vi "OutputDialog.vi"() -> (3 "Cancelled?":bool)   [LabVIEW 2020]
doc: "Use this template to create a dialog box with event handling."
uses:
  global/SettingVariable.vi
  <vilib>/Utility/config.llb/Write Key (Boolean).vi
  <vilib>/Utility/config.llb/Write Key (U32).vi
  <vilib>/Utility/config.llb/Write Key (I32).vi
  <vilib>/Utility/config.llb/Write Key (Double).vi
  <vilib>/Utility/config.llb/NI_LVConfig.lvlib
panel:
  in  "输出电压控件组":T1(array[cluster])=[{"开关"=FALSE, "输出选择"=0, "电压范围"={"Numeric"=5, "Numeric"=1}, "线性/对数"=FALSE, "物理量上限"=100.0, "物理量下限"=-100.0}, {"开关"=FALSE, "输出选择"=0, "电压范围"={"Numeric"=5, "Numeric"=1}, "线性/对数"=FALSE, "物理量上限"=100.0, "物理量下限"=-100.0}, {"开关"=FALSE, "输出选择"=0, "电压范围"={"Numeric"=5, "Numeric"=1}, "线性/对数"=FALSE, "物理量上限"=100.0, "物理量下限"=-100.0}, {"开关"=FALSE, "输出选择"=0, "电压范围"={"Numeric"=5, "Numeric"=1}, "线性/对数"=FALSE, "物理量上限"=100.0, "物理量下限"=-100.0}] {"电压范围" scale=-10.0..10.0; "输出选择" items=["电流1", "电流1反应性", "电流2", "电流2反应性"]}
  out "电流输入指示":bool[](array[boolean])
  out "电压标尺指示":u16[](array[ring]) items=["计数通量", "电压通量", "电流通量", "棒位", "温度", "P2参数", "硼浓度"]
  out "电压输入指示":bool[](array[boolean])
  in  "Cancel":bool
  in  "OK":bool
  # "输入状态"
  # "输出电压设置"
  # "输出电压1："
  # "输出电压2："
  # "输出电压3："
  # "输出电压4："
  # "电流1"
  # "电流2"
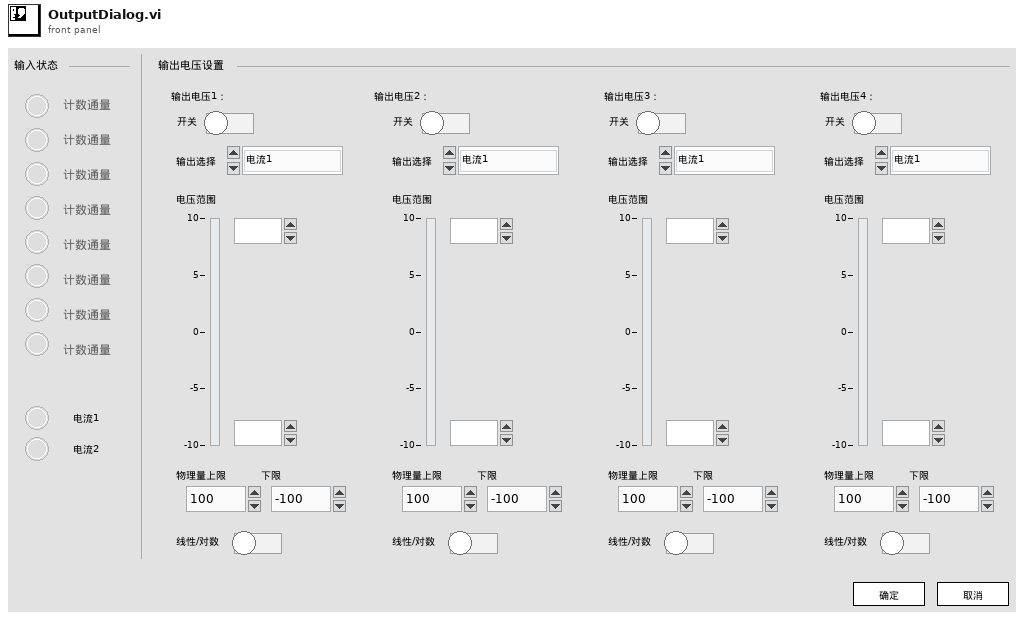
[diagram p1: front panel]
types:
  T1 = cluster{"开关":bool, "输出选择":u16, "电压范围":cluster{"Numeric":i32, "Numeric":i32}, "线性/对数":bool, "物理量上限":dbl, "物理量下限":dbl}[]
  T2 = cluster{"switch":bool, "voltage upper":i32, "voltage lower":i32, "physics upper":dbl, "physics lower":dbl, "input":u16, "log":bool}[]
  T3 = cluster{"switch":bool, "name":string, "voltage upper":i32, "voltage lower":i32, "physics upper":dbl, "physics lower":dbl, "scale":u16}[]
  T4 = cluster{"开关":bool, "输出选择":u16, "电压范围":cluster{"Numeric":i32, "Numeric":i32}, "线性/对数":bool, "物理量上限":dbl, "物理量下限":dbl}
  T5 = enum16{"fractional", "engineering", "exponential"}
  T6 = typedef "NI_LVConfig.lvlib/Config Data RefNum.ctl" = refnum<k1>
  T7 = cluster{"switch":bool, "voltage upper":i32, "voltage lower":i32, "physics upper":dbl, "physics lower":dbl, "input":u16, "log":bool}
  T8 = cluster{"开关":bool, "输出选择":bool, "电压范围":cluster{"Numeric":bool, "Numeric":bool}, "线性/对数":bool, "物理量上限":bool, "物理量下限":bool}[]
  T9 = enum32{"Bad", "Idle", "Run top level", "Running"}
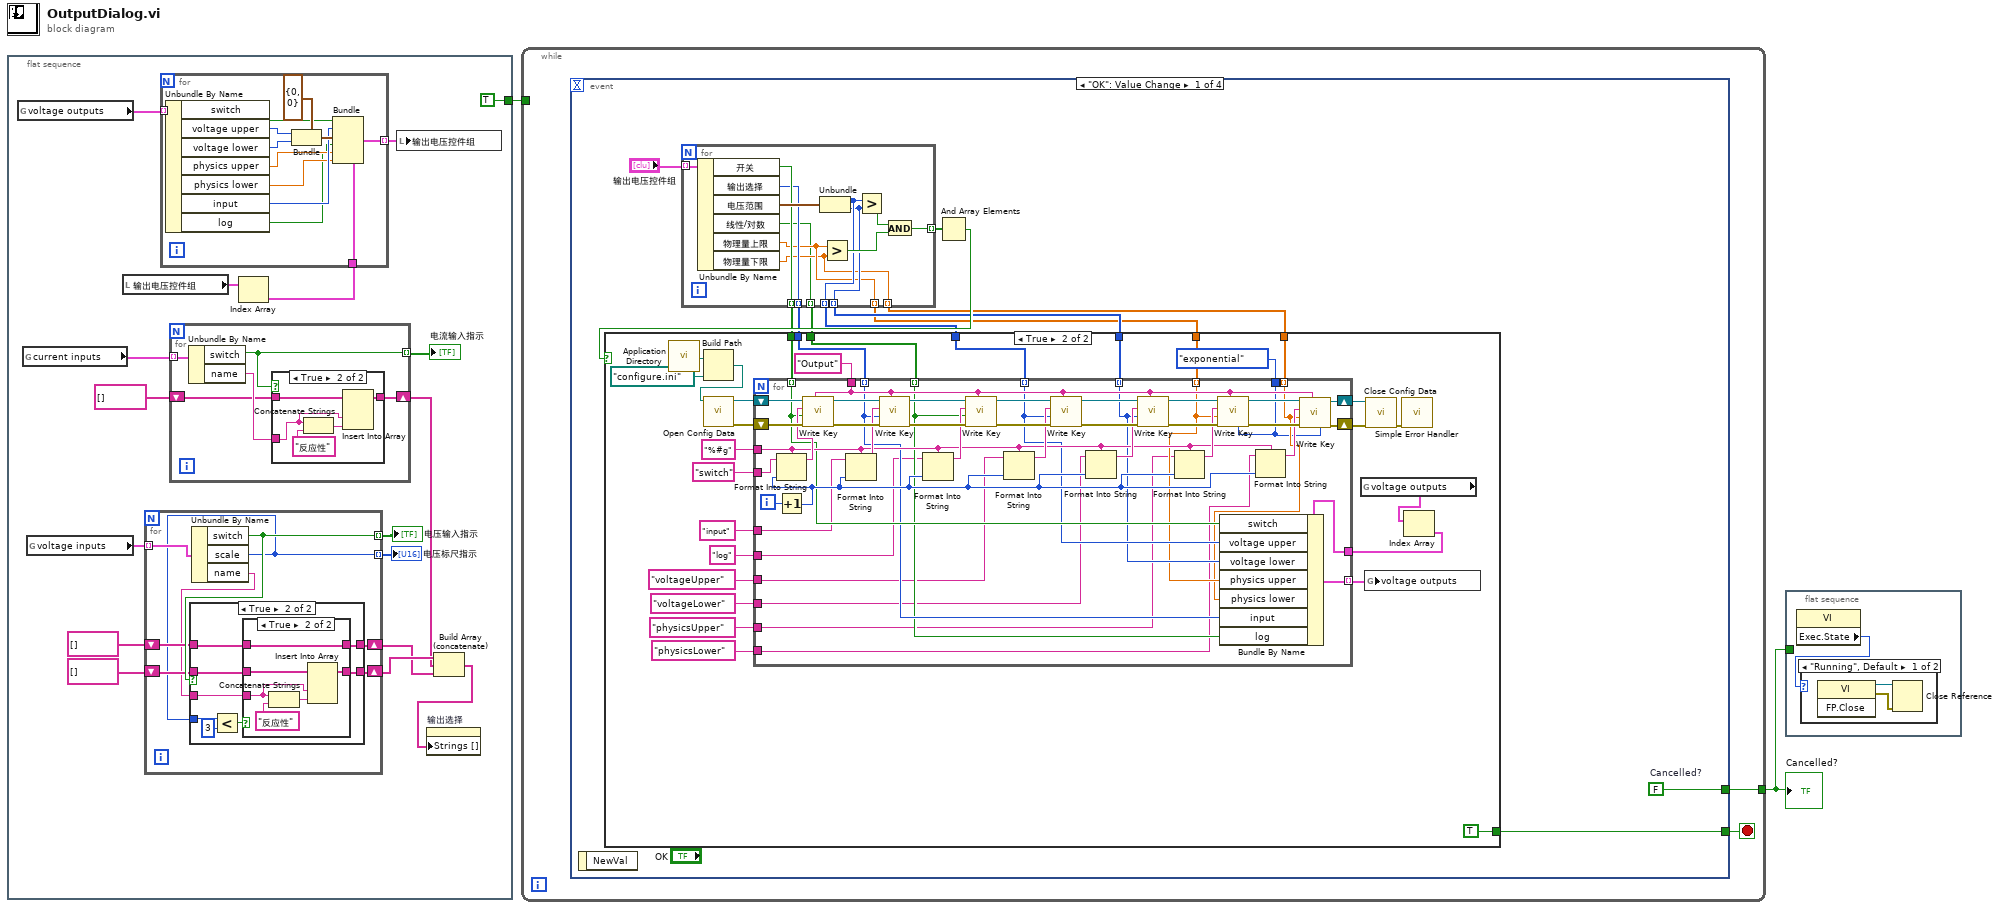
[diagram p0: block diagram]
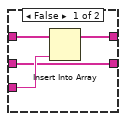
[diagram p4: hidden frame]
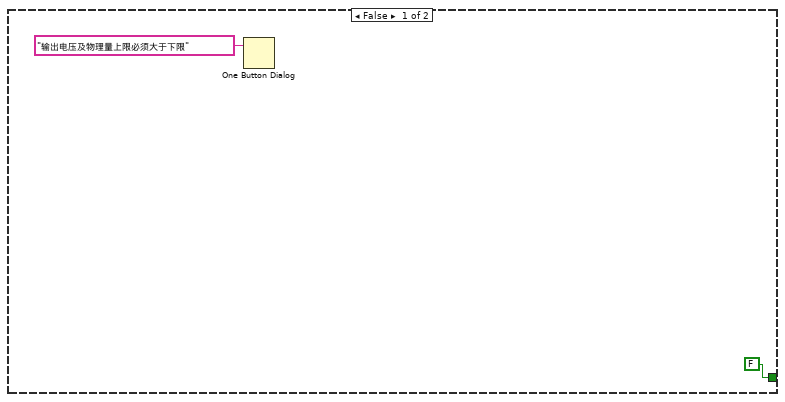
[diagram p6: hidden frame]
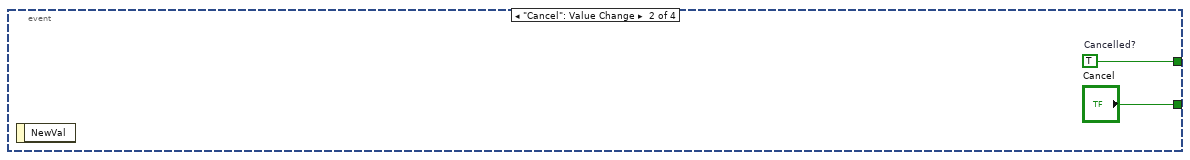
[diagram p7: hidden frame]
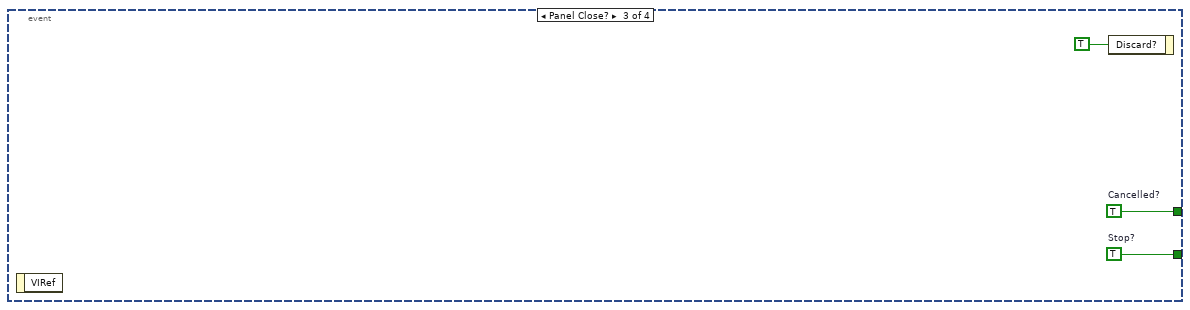
[diagram p8: hidden frame]
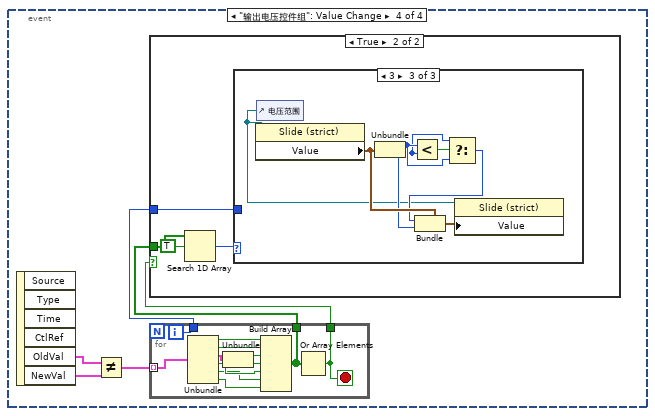
[diagram p9: hidden frame]
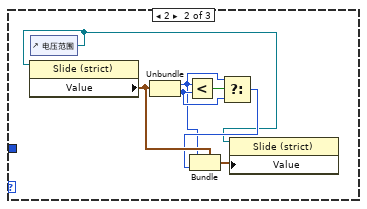
[diagram p12: hidden frame]
diagram:
  n1 = flat-sequence {
    tunnel: [TRUE] -> w2
    frame #0 {
      n2 = global read "SettingVariable.vi" "voltage outputs"() -> (w14:T2)
      n3 = global read "SettingVariable.vi" "current inputs"() -> (w19:cluster{"name":string, "switch":bool}[])
      n4 = global read "SettingVariable.vi" "voltage inputs"() -> (w17:T3)
      n5 = local read "输出电压控件组"() -> (w13:T1)
      n6 = for {
        tunnel: w17 -> [w39] mode=indexing
        tunnel: [w38] -> w16 mode=indexing
        tunnel: [w32] -> w15 mode=indexing
        shift-right: [w36] -> w6
        shift-left: string[] [] ("子数组") -> [w37]
        shift-right: [w34] -> w4
        shift-left: string[] [] ("子数组") -> [w35]
        n7 = Unbundle By Name(w39) -> ("switch"=w38:bool, "scale"=w32:u16, "name"=w33:string)
        n8 = case shown="True" w38 {
          tunnel: w37 -> [w41 w46]
          tunnel: w32 -> [_ w49]
          tunnel: [w41 w45] -> w36
          tunnel: w33 -> [_ w44]
          tunnel: w35 -> [w40 w42]
          tunnel: [w40 w43] -> w34
          frame False {
          }
          frame True {
            n9 = Less?(x=w49, y=u16 3) -> (x < y?=w47:bool)
            n10 = case shown="True" w47 {
              tunnel: w46 -> [w50 w57]
              tunnel: [w50 w56] -> w45
              tunnel: w44 -> [w53 w55]
              tunnel: [w51 w54] -> w43
              tunnel: w42 -> [w52 w54]
              frame False {
                n11 = Insert Into Array(array=w52, new element=w53) -> (w51:string[])  [unwired: 1 in]
              }
              frame True {
                n12 = Concatenate Strings(w55, "反应性" ("字符串")) -> (w58:string)
                n13 = Insert Into Array(array=w57, new element #1=w55, new element #2=w58) -> (w56:string[])  [unwired: 1 in]
              }
            }
          }
        }
      }
      "电压输入指示" <- w16
      "电压标尺指示" <- w15
      n14 = for {
        tunnel: w19 -> [w64] mode=indexing
        tunnel: [w63] -> w18 mode=indexing
        shift-right: [w61] -> w5
        shift-left: string[] [] -> [w60]
        n15 = Unbundle By Name(w64) -> ("switch"=w63:bool, "name"=w62:string)
        n16 = case shown="True" w63 {
          tunnel: w60 -> [w65 w70]
          tunnel: [w65 w69] -> w61
          tunnel: w62 -> [_ w66]
          frame False {
          }
          frame True {
            n17 = Concatenate Strings(w66, "反应性" ("字符串")) -> (w67:string)
            n18 = Insert Into Array(array=w70, new element #1=w66, new element #2=w67) -> (w69:string[])  [unwired: 1 in]
          }
        }
      }
      "电流输入指示" <- w18
      n19 = Index Array(array=w13) -> (element=w12:T4)  [unwired: 1 in]
      n20 = for {
        tunnel: w14 -> [w31] mode=indexing
        tunnel: w12 -> [w27]
        tunnel: [w20] -> w11 mode=indexing
        n21 = Unbundle By Name(w31) -> ("switch"=w24:bool, "voltage upper"=w29:i32, "voltage lower"=w28:i32, "physics upper"=w23:dbl, "physics lower"=w22:dbl, "input"=w25:u16, "log"=w21:bool)
        n22 = Bundle(cluster=cluster{i32, i32} {0, 0}, w29, w28) -> (w26:cluster{i32, i32})
        n23 = Bundle(cluster=w27, "开关"=w24, "输出选择"=w25, "电压范围"=w26, "线性/对数"=w21, "物理量上限"=w23, "物理量下限"=w22) -> (w20:T4)
      }
      n24 = local write "输出电压控件组"(w11) -> ()
      n25 = Build Array (concatenate)(w6, w5, w4) -> (w3:string[])
      n26 = property on="输出选择" class="Ring (strict)"("Strings []"=w3) -> ()  [unwired: 2 in, 2 out]
    }
  }
  n27 = while {
    tunnel: [w71] -> w1
    tunnel: w2 -> [_]
    stop <- w72 stop-if-true
    n28 = event shown="[0] \"OK\": Value Change" {
      selector: _ -> [_ _ _ _]
      dyn-events: _ -> [_ _ _ _]
      timeout: _ -> [_ _ _ _]
      tunnel: [w73 "Cancel" w175 _] -> w72
      tunnel: [w84 w173 w174 _] -> w71
      event "OK": Value Change {
        w84 = FALSE  # Cancelled?
        n29 = event-data() -> ()  [unwired: 1 in, 1 out]
        n30 = for {
          tunnel: "输出电压控件组" -> [w171] mode=indexing
          tunnel: [w167] -> w82 mode=indexing
          tunnel: [w166] -> w80 mode=indexing
          tunnel: [w165] -> w79 mode=indexing
          tunnel: [w164] -> w77 mode=indexing
          tunnel: [w163] -> w76 mode=indexing
          tunnel: [w162] -> w75 mode=indexing
          tunnel: [w161] -> w74 mode=indexing
          tunnel: [w160] -> w78 mode=indexing
          n31 = Unbundle By Name(w171) -> ("开关"=w166:bool, "输出选择"=w165:u16, "电压范围"=w170:cluster{"Numeric":i32, "Numeric":i32}, "线性/对数"=w160:bool, "物理量上限"=w162:dbl, "物理量下限"=w161:dbl)
          n32 = Unbundle(w170) -> ("Numeric"=w164:i32, "Numeric"=w163:i32)
          n33 = Greater?(x=w162, y=w161) -> (0:w168:bool)
          n34 = Greater?(x=w164, y=w163) -> (0:w169:bool)
          n35 = And(x=w169, y=w168) -> (x .and. y?=w167:bool)
        }
        n36 = And Array Elements(Boolean array=w82) -> (logical AND=w81:bool)
        n37 = case shown="True" w81 {
          tunnel: w80 -> [_ w115]
          tunnel: w79 -> [_ w103]
          tunnel: w78 -> [_ w102]
          tunnel: w77 -> [_ w101]
          tunnel: w76 -> [_ w100]
          tunnel: w75 -> [_ w99]
          tunnel: w74 -> [_ w98]
          tunnel: [FALSE ("Stop?") TRUE ("Stop?")] -> w73
          frame False {
            n38 = One Button Dialog(message="输出电压及物理量上限必须大于下限") -> ()  [unwired: 1 in, 1 out]
          }
          frame True {
            n39 = call <vilib>:"Application Directory.vi"() -> ("Application Directory"=w114:path)
            n40 = Build Path(base path=w114, name or relative path=path "configure.ini") -> (appended path=w112:path)
            n41 = call <vilib>:"Open Config Data.vi"("configuration file path"=w112) -> ("error out"=w110:errorcluster, "refnum"=w111:T6)  [unwired: 2 in, 7 out]
            n42 = global read "SettingVariable.vi" "voltage outputs"() -> (w96:T2)
            n43 = Index Array(array=w96) -> (element=w95:T7)  [unwired: 1 in]
            n44 = for {
              tunnel: w115 -> [w129] mode=indexing
              tunnel: "Output" ("section") -> [w137]
              tunnel: "%#g" ("section") -> [w132]
              tunnel: "switch" ("initial string") -> [w156]
              shift-right: [w142] -> w104
              shift-left: w110 -> [w158]
              shift-right: [w143] -> w105
              shift-left: w111 -> [w159]
              tunnel: w103 -> [w128] mode=indexing
              tunnel: w102 -> [w127] mode=indexing
              tunnel: w101 -> [w126] mode=indexing
              tunnel: w100 -> [w125] mode=indexing
              tunnel: w99 -> [w124] mode=indexing
              tunnel: w98 -> [w123] mode=indexing
              tunnel: [w131] -> w97 mode=indexing
              tunnel: w95 -> [w130]
              tunnel: "input" ("initial string") -> [w122]
              tunnel: "log" ("initial string") -> [w121]
              tunnel: "voltageUpper" ("initial string") -> [w120]
              tunnel: "voltageLower" ("initial string") -> [w119]
              tunnel: "physicsUpper" ("initial string") -> [w118]
              tunnel: "physicsLower" ("initial string") -> [w117]
              tunnel: T5."exponential" ("format (fractional)") -> [w116]
              i -> [w157]
              n45 = Increment(x=w157) -> (x+1=w133:i32)
              n46 = Format Into String(format string=w132, initial string=w156, w133) -> (resulting string=w155:string)  [unwired: 1 in, 1 out]
              n47 = call-poly <vilib>:"Write Key.vi"("section"=w137, "error in (no error)"=w158, "value"=w129, "key"=w155, "refnum"=w159) -> ("error out"=w154:errorcluster, "refnum out"=w153:T6)  [unwired: 4 in, 1 out]
              n48 = Format Into String(format string=w132, initial string=w122, w133) -> (resulting string=w148:string)  [unwired: 1 in, 1 out]
              n49 = call-poly <vilib>:"Write Key.vi"("section"=w137, "error in (no error)"=w154, "value"=w128, "key"=w148, "refnum"=w153) -> ("error out"=w151:errorcluster, "refnum out"=w152:T6)  [unwired: 4 in, 1 out]
              n50 = Format Into String(format string=w132, initial string=w121, w133) -> (resulting string=w147:string)  [unwired: 1 in, 1 out]
              n51 = call-poly <vilib>:"Write Key.vi"("section"=w137, "error in (no error)"=w151, "value"=w127, "key"=w147, "refnum"=w152) -> ("error out"=w149:errorcluster, "refnum out"=w150:T6)  [unwired: 4 in, 1 out]
              n52 = Format Into String(format string=w132, initial string=w120, w133) -> (resulting string=w146:string)  [unwired: 1 in, 1 out]
              n53 = call-poly <vilib>:"Write Key.vi"("section"=w137, "error in (no error)"=w149, "value"=w126, "key"=w146, "refnum"=w150) -> ("error out"=w144:errorcluster, "refnum out"=w145:T6)  [unwired: 4 in, 1 out]
              n54 = Format Into String(format string=w132, initial string=w119, w133) -> (resulting string=w136:string)  [unwired: 1 in, 1 out]
              n55 = call-poly <vilib>:"Write Key.vi"("section"=w137, "error in (no error)"=w144, "value"=w125, "key"=w136, "refnum"=w145) -> ("error out"=w141:errorcluster, "refnum out"=w138:T6)  [unwired: 4 in, 1 out]
              n56 = Format Into String(format string=w132, initial string=w118, w133) -> (resulting string=w135:string)  [unwired: 1 in, 1 out]
              n57 = call-poly <vilib>:"Write Key.vi"("format (fractional)"=w116, "section"=w137, "error in (no error)"=w141, "value"=w124, "key"=w135, "refnum"=w138) -> ("error out"=w140:errorcluster, "refnum out"=w139:T6)  [unwired: 3 in, 1 out]
              n58 = Bundle By Name(cluster=w130, "switch"=w129, "voltage upper"=w126, "voltage lower"=w125, "physics upper"=w124, "physics lower"=w123, "input"=w128, "log"=w127) -> (w131:T7)
              n59 = Format Into String(format string=w132, initial string=w117, w133) -> (resulting string=w134:string)  [unwired: 1 in, 1 out]
              n60 = call-poly <vilib>:"Write Key.vi"("format (fractional)"=w116, "section"=w137, "error in (no error)"=w140, "value"=w123, "key"=w134, "refnum"=w139) -> ("error out"=w142:errorcluster, "refnum out"=w143:T6)  [unwired: 3 in, 1 out]
            }
            n61 = global write "SettingVariable.vi" "voltage outputs"(w97) -> ()
            n62 = call <vilib>:"Close Config Data.vi"("error in (no error)"=w104, "refnum"=w105) -> ("error out"=w106:errorcluster)  [unwired: 1 in, 8 out]
            n63 = call <vilib>:"Simple Error Handler.vi"("error in (no error)"=w106) -> ()  [unwired: 1 in, 8 out]
          }
        }
      }
      event "Cancel": Value Change {
        w173 = TRUE  # Cancelled?
        n64 = event-data() -> ()  [unwired: 1 in, 1 out]
      }
      event Panel Close? {
        w174 = TRUE  # Cancelled?
        w175 = TRUE  # Stop?
        n65 = event-data() -> ()  [unwired: 1 in, 1 out]
        n66 = event-data("Discard?"=TRUE) -> ()  [unwired: 1 in, 1 out]
      }
      event "输出电压控件组": Value Change {
        n67 = event-data() -> ("OldVal"=w182:T1, "NewVal"=w177:T1)  [unwired: 1 in, 4 out]
        n68 = Not Equal?(x=w182, y=w177) -> (x != y?=w181:T8)
        n69 = for {
          tunnel: w181 -> [w212] mode=indexing
          tunnel: [w203] -> w180
          tunnel: [w202] -> w179
          tunnel: [w201] -> w178
          i -> [w201]
          stop <- w203 stop-if-true
          n70 = Unbundle(w212) -> ("开关"=w211:bool, "输出选择"=w209:bool, "电压范围"=w210:cluster{"Numeric":bool, "Numeric":bool}, "线性/对数"=w206:bool, "物理量上限"=w205:bool, "物理量下限"=w204:bool)
          n71 = Unbundle(w210) -> ("Numeric"=w208:bool, "Numeric"=w207:bool)
          n72 = Build Array(w211, w209, w208, w207, w206, w205, w204) -> (w202:bool[])
          n73 = Or Array Elements(Boolean array=w202) -> (logical OR=w203:bool)
        }
        n74 = case shown="True" w180 {
          tunnel: w179 -> [_ w186]
          tunnel: w178 -> [_ w183]
          frame False {
          }
          frame True {
            n75 = Search 1D Array(1D array=w186, element=TRUE) -> (index of element=w184:i32)  [unwired: 1 in]
            n76 = case shown="3" w184 {
              tunnel: w183 -> [_ _ _]
              frame 0, Default {
              }
              frame 2 {
                n77 = control-ref of="电压范围"() -> (w187:refnum<vi>)
                n78 = property class="Slide (strict)"(reference=w187) -> ("Value"=w190:cluster{"Numeric":i32, "Numeric":i32})  [unwired: 1 in, 2 out]
                n79 = Unbundle(w190) -> ("Numeric"=w188:i32, "Numeric"=w193:i32)
                n80 = Less?(x=w188, y=w193) -> (x < y?=w192:bool)
                n81 = Select(t=w188, s=w192, f=w193) -> (s? t:f=w189:i32)
                n82 = Bundle(cluster=w190, "Numeric"=w188, "Numeric"=w189) -> (w191:cluster{"Numeric":i32, "Numeric":i32})
                n83 = property class="Slide (strict)"(reference=w187, "Value"=w191) -> ()  [unwired: 1 in, 2 out]
              }
              frame 3 {
                n84 = control-ref of="电压范围"() -> (w194:refnum<vi>)
                n85 = property class="Slide (strict)"(reference=w194) -> ("Value"=w198:cluster{"Numeric":i32, "Numeric":i32})  [unwired: 1 in, 2 out]
                n86 = Unbundle(w198) -> ("Numeric"=w196:i32, "Numeric"=w195:i32)
                n87 = Less?(x=w196, y=w195) -> (x < y?=w200:bool)
                n88 = Select(t=w195, s=w200, f=w196) -> (s? t:f=w197:i32)
                n89 = Bundle(cluster=w198, "Numeric"=w197, "Numeric"=w195) -> (w199:cluster{"Numeric":i32, "Numeric":i32})
                n90 = property class="Slide (strict)"(reference=w194, "Value"=w199) -> ()  [unwired: 1 in, 2 out]
              }
            }
          }
        }
      }
    }
  }
  "Cancelled?" <- w1
  n91 = flat-sequence {
    tunnel: w1 -> [_]
    frame #0 {
      n92 = property class="VI"() -> ("Exec.State"=w213:T9)  [unwired: 2 in, 2 out]
      n93 = case shown="\"Running\", Default" w213 {
        frame "Running", Default {
          n94 = invoke class="VI" method="FP.Close"() -> (reference out=w214:refnum<vi>, error out=w215:errorcluster)  [unwired: 3 in, 1 out]
          n95 = Close Reference(reference=w214, error in (no error)=w215) -> ()  [unwired: 1 out]
        }
        frame "Run top level" {
        }
      }
    }
  }
